vi "未命名 1.vi"() -> ()   [LabVIEW 2015]
uses:
  <vilib>/vision/Contour.llb/IMAQ Contour Curve Extraction.ctl
  <vilib>/vision/Contour.llb/IMAQ Connect Range Setting.ctl
panel:
  in  "Match Mode (Contour Analysis 1)":T1
  in  "Curve Extraction 2 (Contour Analysis 1)":T2={"Extraction Mode"=0, "Edge Threshold"=75, "Edge Filter Size"=2, "Min Length"=25, "Search Step Size"=15, "Max Endpoint Gap"=10, "Subpixel"=TRUE} {"Extraction Mode" items=["Normal", "Uniform Regions"]; "Edge Filter Size" items=["Fine", "Normal", "Contour Tracing"]; "Max Endpoint Gap" min=0; "Search Step Size" min=1 max=255 step=1; "Min Length" min=0; "Edge Threshold" min=1 max=350 step=1}
  in  "Curve Connection (Contour Analysis 1)":T3[](array[typedef])=[{"Match Constraints"=0, "Min"=1.0, "Max"=12.0}] {"Max" format="%.2f"; "Min" format="%.2f"; "Match Constraints" items=["Distance (pixel)", "Angle Difference (degrees)", "Connectivity Distance (pixel)", "Gradient Difference (degrees)"]}
  in  "Contour Selection (Contour Analysis 1)":T4(ring)=enum."Maximum Length"
  in  "Search Direction (Contour Analysis 1)":T5(ring)=enum."Annulus Inner To Outer"
  in  "Curve Extraction (Contour Analysis 1)":T2={"Extraction Mode"=0, "Edge Threshold"=75, "Edge Filter Size"=2, "Min Length"=25, "Search Step Size"=15, "Max Endpoint Gap"=10, "Subpixel"=TRUE} {"Extraction Mode" items=["Normal", "Uniform Regions"]; "Edge Filter Size" items=["Fine", "Normal", "Contour Tracing"]; "Max Endpoint Gap" min=0; "Search Step Size" min=1 max=255 step=1; "Min Length" min=0; "Edge Threshold" min=1 max=350 step=1}
  out "Image":T6(plugin-control)
  in  "File Path":path
  # "Range"
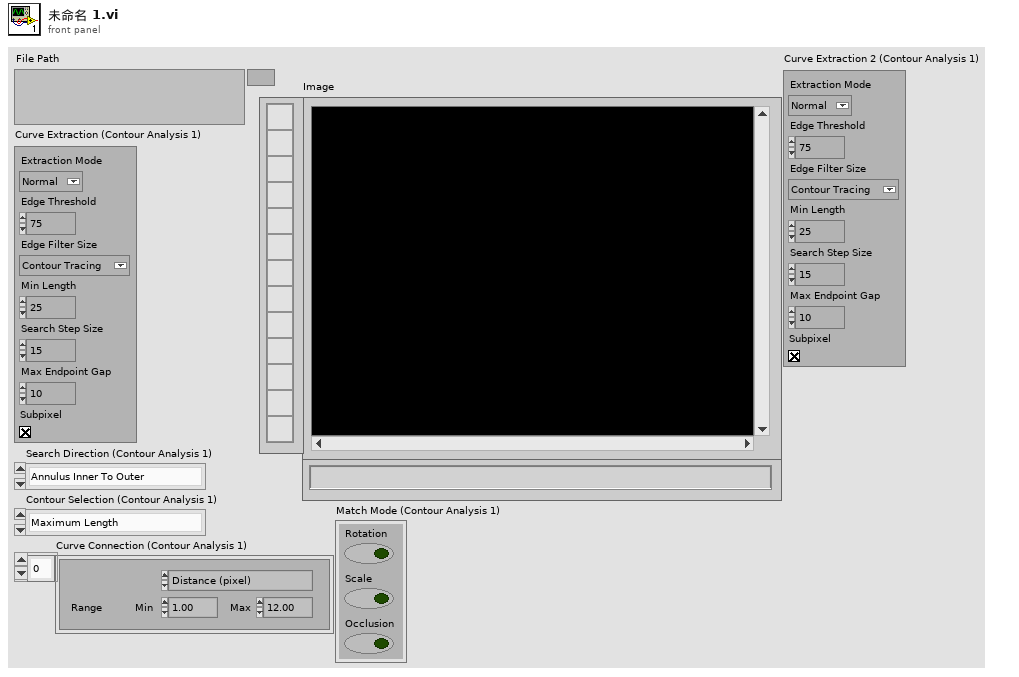
[diagram p1: front panel]
types:
  T1 = cluster{"Rotation":bool, "Scale":bool, "Occlusion":bool}
  T2 = typedef "IMAQ Contour Curve Extraction.ctl" = cluster{"Extraction Mode":u32, "Edge Threshold":i32, "Edge Filter Size":u32, "Min Length":i32, "Search Step Size":i32, "Max Endpoint Gap":i32, "Subpixel":bool}
  T3 = typedef "IMAQ Connect Range Setting.ctl" = cluster{"Match Constraints":u32, "Min":dbl, "Max":dbl}
  T4 = enum16{"Closest To Search Start", "Maximum Length", "Strongest Mean Gradient Change"}
  T5 = enum16{"Rect Left To Right", "Rect Right To Left", "Rect Top To Bottom", "Rect Bottom To Top", "Annulus Inner To Outer", "Annulus Outer To Inner", "Annulus Start Angle To End Angle", "Annulus End Angle To Start Angle"}
  T6 = typedef "IMAQ Image.ctl" = refnum<image>
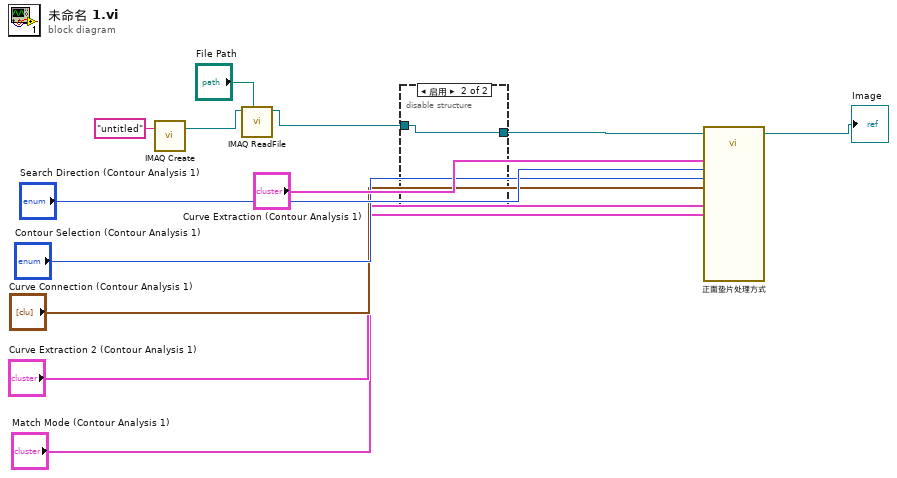
[diagram p0: block diagram]
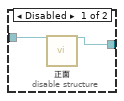
[diagram p2: hidden frame]
diagram:
  n1 = call "IMAQ Create"("Image Name"="untitled") -> ("New Image"=w11:T6)  [unwired: 4 in, 1 out]
  n2 = call "IMAQ ReadFile"("File Path"="File Path", "Image"=w11) -> ("Image Out"=w9:T6)  [unwired: 5 in, 4 out]
  n3 = disable-structure shown="启用" {
    disable-tunnel: w9 -> [w14 w15]
    disable-tunnel: [w13 w15] -> w8
    frame Disabled {
      n4 = call "正面"("Image In"=w14) -> ("Image Out"=w13:T6)  [unwired: 25 in, 1 out]
    }
    frame Enabled {
    }
  }
  n5 = call "正面垫片处理方式"("Image In"=w8, "Curve Extraction (Contour Analysis 1)"="Curve Extraction (Contour Analysis 1)", "Search Direction (Contour Analysis 1)"="Search Direction (Contour Analysis 1)", "Contour Selection (Contour Analysis 1)"="Contour Selection (Contour Analysis 1)", "Curve Connection (Contour Analysis 1)"="Curve Connection (Contour Analysis 1)", "Curve Extraction 2 (Contour Analysis 1)"="Curve Extraction 2 (Contour Analysis 1)", "Match Mode (Contour Analysis 1)"="Match Mode (Contour Analysis 1)") -> ("Image Out"=→"Image":T6)  [unwired: 13 in, 7 out]
